vi "Run Continuous Capture Demonstration.vi"() -> ()   [LabVIEW 2017]
doc: "Run a demonstration using a device driver, with the data shared across a local network.\n\nUses a configurable GUI, with multiple tabs and active plots."
uses:
  Communications/Typedefs/Data Size--Enum.ctl
  SubVIs/API - Continuous Capture - Capture Continuously.vi
  GUI/Plots/Plot Data - Main GUI.vi
  GUI/Plots/DTacq Plot Display Library.lvlib
  DTACQ - Network Enabled Device Driver.lvlib
  Communications/Communications Library.lvlib
panel:
  in  "Start Button":bool
  in  "Data Size":T1
  in  "Buffer Block Size (Samples/Channel)":i32=1000
  in  "Maximum Capture Rate (Full Buffers/Second)":i32=100
  in  "Configuration file path (Leave Blank for Defaults)":path
  # "Continuous Capture"
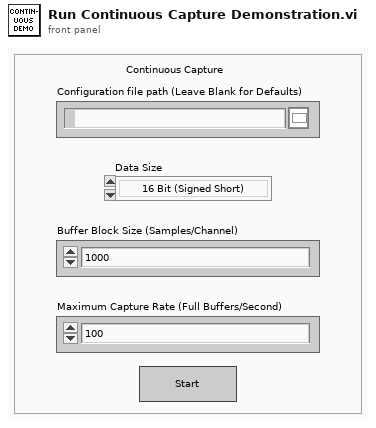
[diagram p1: front panel]
types:
  T1 = typedef "Communications Library.lvlib/Data Size--Enum.ctl" = enum16{"16 Bit (Signed Short)", "32 Bit (Signed Long)"}
  T2 = enum32{"Invalid", "Standard", "Closed", "Hidden", "Minimized", "Maximized"}
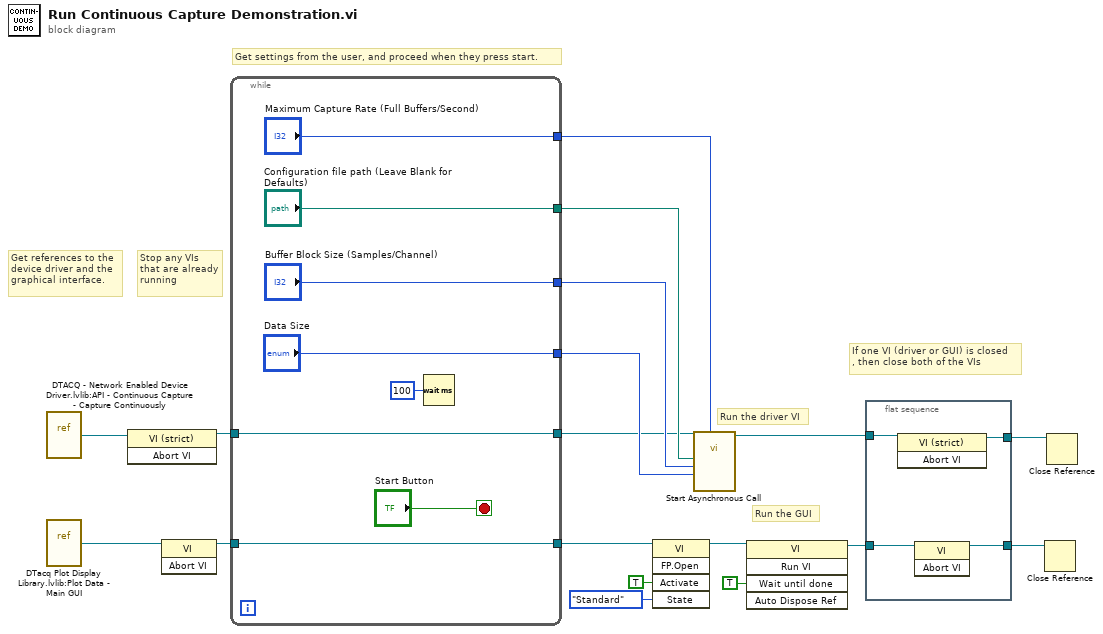
[diagram p0: block diagram]
diagram:
  # "If one VI (driver or GUI) is closed\n, then close both of the VIs"
  # "Run the GUI"
  # "Run the driver VI"
  # "Get settings from the user, and proceed when they press start."
  # "Stop any VIs\nthat are already\nrunning"
  # "Get references to the\ndevice driver and the\ngraphical interface."
  n1 = vi-ref "DTACQ - Network Enabled Device Driver.lvlib:API - Continuous Capture - Capture Continuously.vi"() -> (w16:refnum<vi>)
  n2 = vi-ref "DTacq Plot Display Library.lvlib:Plot Data - Main GUI.vi"() -> (w15:refnum<vi>)
  n3 = invoke class="VI (strict)" method="Abort VI"(reference=w16) -> (reference out=w4:refnum<vi>)  [unwired: 2 in, 2 out]
  n4 = invoke class="VI" method="Abort VI"(reference=w15) -> (reference out=w2:refnum<vi>)  [unwired: 2 in, 2 out]
  n5 = while {
    tunnel: ["Maximum Capture Rate (Full Buffers/Second)"] -> w8
    tunnel: ["Configuration file path (Leave Blank for Defaults)"] -> w7
    tunnel: ["Buffer Block Size (Samples/Channel)"] -> w6
    tunnel: ["Data Size"] -> w5
    tunnel: w4 -> [w22]
    tunnel: [w22] -> w3
    tunnel: w2 -> [w21]
    tunnel: [w21] -> w1
    stop <- "Start Button" stop-if-true
    n6 = Wait (ms)(milliseconds to wait=u32 100) -> ()  [unwired: 1 out]
  }
  n7 = invoke class="VI" method="FP.Open"(reference=w1, "Activate"=TRUE ("Activate?"), "State"=T2."Standard") -> (reference out=w14:refnum<vi>)  [unwired: 2 in, 4 out]
  n8 = call-by-ref "Start Asynchronous Call"(reference=w3, "Maximum Caputre Rate (Full Buffers/Second)"=w8, "Data Size"=w5, "Buffer Block Size (Samples/Channel)"=w6, "Configuration file path"=w7) -> (reference out=w9:refnum<vi>)  [unwired: 8 in, 2 out]
  n9 = invoke class="VI" method="Run VI"(reference=w14, "Wait until done"=TRUE ("Wait Until Done")) -> (reference out=w12:refnum<vi>)  [unwired: 3 in, 4 out]
  n10 = flat-sequence {
    tunnel: w9 -> [w30]
    tunnel: w12 -> [w29]
    tunnel: [w28] -> w11
    tunnel: [w27] -> w10
    frame #0 {
      n11 = invoke class="VI (strict)" method="Abort VI"(reference=w30) -> (reference out=w27:refnum<vi>)  [unwired: 2 in, 2 out]
      n12 = invoke class="VI" method="Abort VI"(reference=w29) -> (reference out=w28:refnum<vi>)  [unwired: 2 in, 2 out]
    }
  }
  n13 = Close Reference(reference=w11) -> ()  [unwired: 1 in, 1 out]
  n14 = Close Reference(reference=w10) -> ()  [unwired: 1 in, 1 out]
